vi "CTRE_Phoenix_CANcoder_ConfigVelocityMeasurementWindow.vi"(6 "timeoutMs":i32, 8 "error in":errorcluster, 10 "windowSize":i32=1, 11 "CTRE_CANcoder_DeviceRef":T1) -> (0 "error out":errorcluster, 3 "CTRE_CANcoder_DeviceRef":T1)   [LabVIEW 2020]
doc: "Sets the number of velocity samples used in the rolling average velocity measurement.\n\n<b>windowSize</b> Number of samples in the rolling average of velocity measurement. Valid values are 1,2,4,8,16,32. If another value is specified, it will truncate to nearest support value.\n<b>timeoutMs</b> Timeout value in ms. If nonzero, function will wait for config success and report an error if it times out. If zero, no blocking or checking is performed."
uses:
  <vilib>/Rock Robotics/WPI/ThirdParty/Phoenix-LabVIEW/CANCoder/Controls/CTRE_Phoenix_CANcoder_DeviceRef.ctl
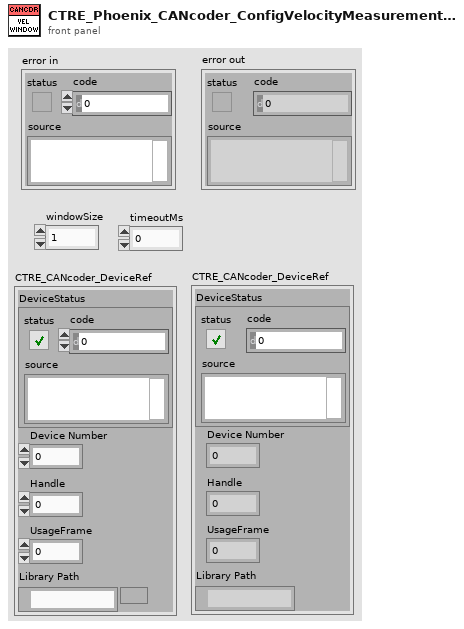
[diagram p1: front panel]
types:
  T1 = typedef "CTRE_Phoenix_CANcoder_DeviceRef.ctl" = cluster{"DeviceStatus":errorcluster, "Device Number":u8, "Handle":u64, "UsageFrame":u32, "Library Path":path}
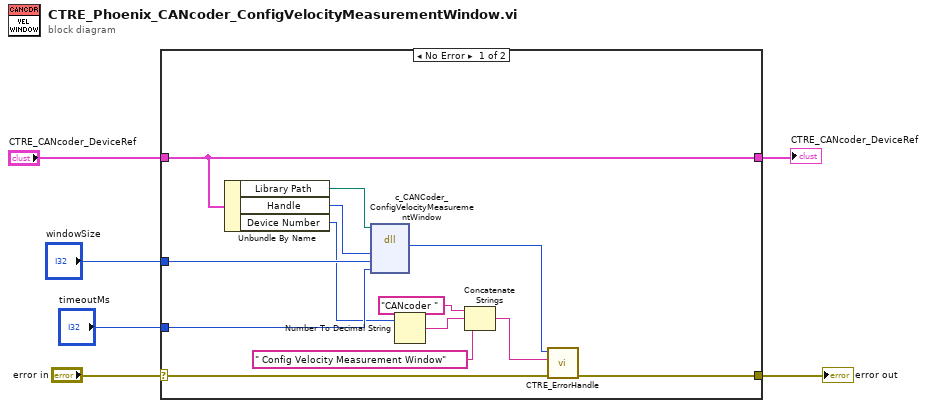
[diagram p0: block diagram]
diagram:
  n1 = case shown="No Error" "error in" {
    selector: "error in" -> [w16 w21]
    tunnel: "CTRE_CANcoder_DeviceRef" -> [w17 w20]
    tunnel: [w15 w21] -> w5
    tunnel: [w17 w20] -> w1
    tunnel: "timeoutMs" -> [w13 _]
    tunnel: "windowSize" -> [w12 _]
    frame No Error {
      n2 = Unbundle By Name(w17) -> ("Library Path"=w19:path, "Handle"=w18:u64, "Device Number"=w7:u8)
      n3 = dll-call lib="?" fn="c_CANCoder_ConfigVelocityMeasurementWindow"(path in=w19, "handle"=w18, "window"=w12, "timeoutMs"=w13) -> ("CTR_Code"=w14:i8)  [unwired: 5 in, 2 out]
      n4 = Number To Decimal String(number=w7) -> (decimal integer string=w11:string)  [unwired: 1 in]
      n5 = Concatenate Strings("CANcoder " ("string"), w11, " Config Velocity Measurement Window" ("string")) -> (w8:string)
      n6 = call <vilib>:"CTRE_ErrorHandle.vi"("error in"=w16, "origin"=w8, "code"=w14) -> ("error out"=w15:errorcluster)  [unwired: 8 in]
    }
    frame Error {
    }
  }
  "error out" <- w5
  "CTRE_CANcoder_DeviceRef" <- w1
